vi "Get CFG wrapper.vi"(8 "error in (no error)":errorcluster caption="错误输入（无错误）", 10 "dwCanNodeId":u32, 11 "dwDevIndex":u32) -> (0 "error out":errorcluster caption="错误输出", 1 "UIM_MCFG_INFO_OBJ":T1, 2 "UIM_ICFG_INFO_OBJ":T2, 3 "function return":u32)   [LabVIEW 2016, in "UISimCanFunc_wrapper.lvlib"]
doc: "_declspec (dllexport) DWORD GetCFG_wrapper(DWORD dwDevIndex, DWORD dwCanNodeId,\n P_DUMMY_UIM_ICFG_INFO_OBJ pDummyICFGInfoOut, P_DUMMY_UIM_MCFG_INFO_OBJ pDummyMCFGInfo);"
uses:
  <userlib>/UISimCanFunc_wrapper/UISimCanFunc_wrapper.lvlib
  <userlib>/UISimCanFunc_wrapper/ctl/UIM_ICFG_INFO_OBJ.ctl
  <userlib>/UISimCanFunc_wrapper/ctl/UIM_MCFG_INFO_OBJ.ctl
  <userlib>/UISimCanFunc_wrapper/UISimCanFunc_wrapper.dll
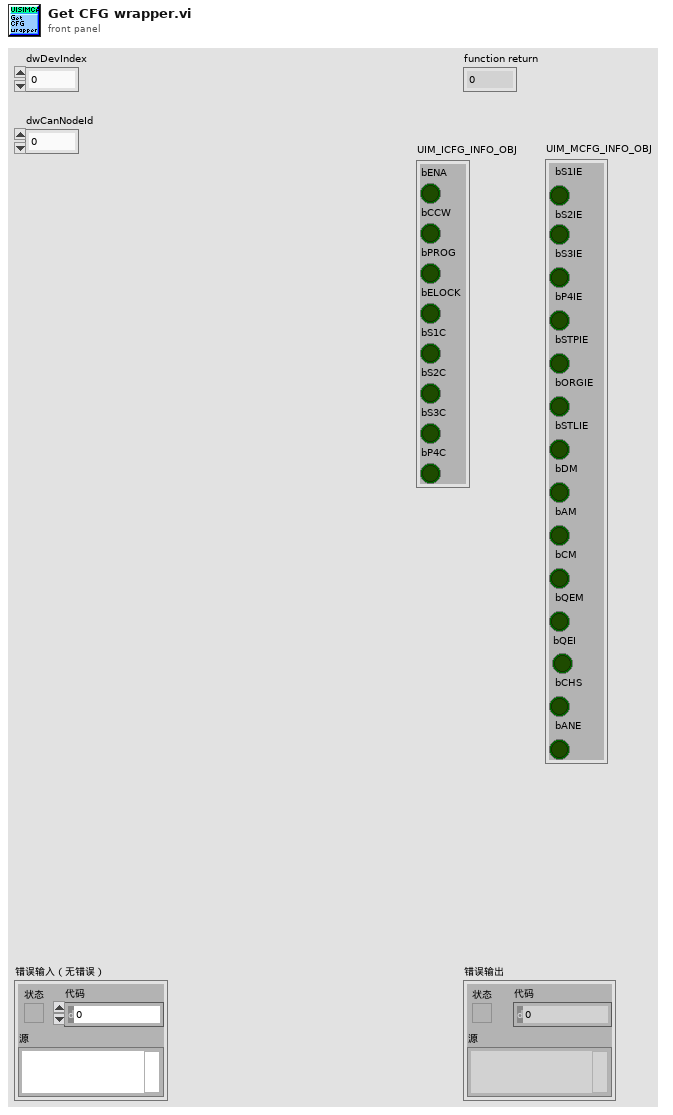
[diagram p1: front panel]
types:
  T1 = typedef "UISimCanFunc_wrapper.lvlib/UIM_MCFG_INFO_OBJ.ctl" = cluster{" bS1IE":bool, " bS2IE":bool, " bS3IE":bool, " bP4IE":bool, " bSTPIE":bool, " bORGIE":bool, " bSTLIE":bool, " bDM":bool, " bAM":bool, " bCM":bool, " bQEM":bool, " bQEI        ":bool, " bCHS":bool, " bANE":bool}
  T2 = typedef "UISimCanFunc_wrapper.lvlib/UIM_ICFG_INFO_OBJ.ctl" = cluster{"bENA":bool, "bCCW":bool, "bPROG":bool, "bELOCK":bool, "bS1C":bool, "bS2C":bool, "bS3C":bool, "bP4C":bool}
  T3 = cluster{"bENA":i32, "bCCW":i32, "bPROG":i32, "bELOCK":i32, "bS1C":i32, "bS2C":i32, "bS3C":i32, "bP4C":i32}
  T4 = cluster{"bS1IE":i32, "bS2IE":i32, "bS3IE":i32, "bP4IE":i32, "bSTPIE":i32, "bORGIE":i32, "bSTLIE":i32, "bDM":i32, "bAM":i32, "bCM":i32, "bQEM":i32, "bQEI":i32, "bCHS":i32, "bANE":i32}
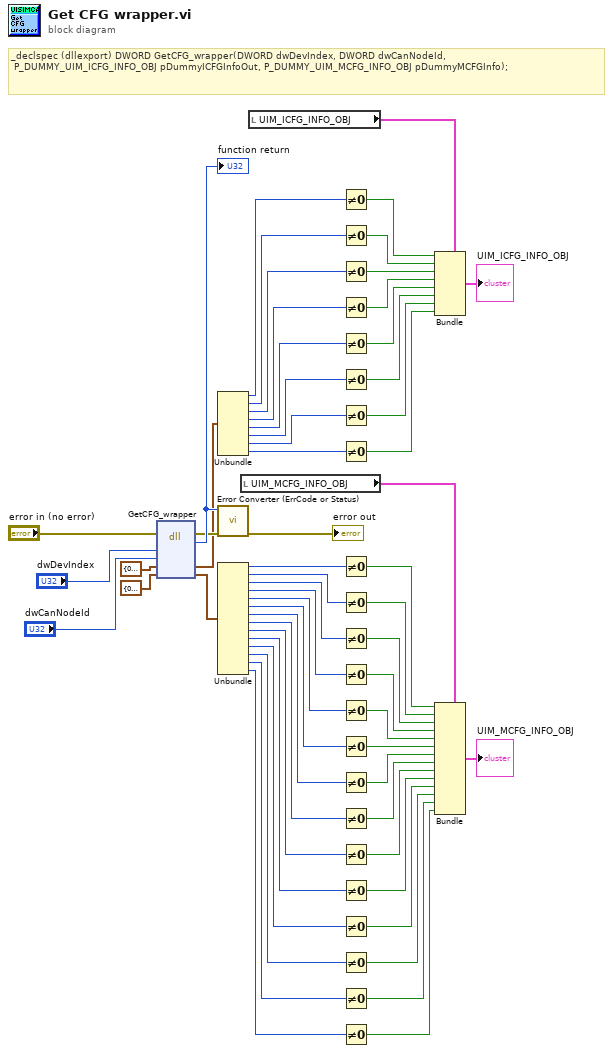
[diagram p0: block diagram]
diagram:
  # "_declspec (dllexport) DWORD GetCFG_wrapper(DWORD dwDevIndex, DWORD dwCanNodeId,\n\tP_DUMMY_UIM_ICFG_INFO_OBJ pDummyICFGInfoOut, P_DUMMY_UIM_MCFG_INFO_OBJ pDummyMCFGInfo);"
  n1 = dll-call lib="C:/Program Files (x86)/National Instruments/LabVIEW 2016/user.lib/UISimCanFunc_wrapper/UISimCanFunc_wrapper.*" fn="GetCFG_wrapper"(error in="error in (no error)", "dwDevIndex"="dwDevIndex", "dwCanNodeId"="dwCanNodeId", "pDummyICFGInfoOut"=T3 {"bENA"=0, "bCCW"=0, "bPROG"=0, "bELOCK"=0, "bS1C"=0, "bS2C"=0, "bS3C"=0, "bP4C"=0}, "pDummyMCFGInfo"=T4 {"bS1IE"=0, "bS2IE"=0, "bS3IE"=0, "bP4IE"=0, "bSTPIE"=0, "bORGIE"=0, "bSTLIE"=0, "bDM"=0, "bAM"=0, "bCM"=0, "bQEM"=0, "bQEI"=0, "bCHS"=0, "bANE"=0}) -> (error out=w54:errorcluster, w58:u32, "pDummyICFGInfoOut"=w1:T3, "pDummyMCFGInfo"=w20:T4)  [unwired: 4 in, 1 out]
  "function return" <- w58
  n2 = Unbundle(w1) -> ("bENA"=w19:i32, "bCCW"=w18:i32, "bPROG"=w17:i32, "bELOCK"=w16:i32, "bS1C"=w11:i32, "bS2C"=w10:i32, "bS3C"=w9:i32, "bP4C"=w8:i32)
  n3 = call <userlib>:"Error Converter (ErrCode or Status).vi"("error in (no error)"=w54, "error code"=w58) -> ("error out"=→"error out":errorcluster)  [unwired: 9 in]
  n4 = Unbundle(w20) -> ("bS1IE"=w50:i32, "bS2IE"=w49:i32, "bS3IE"=w48:i32, "bP4IE"=w47:i32, "bSTPIE"=w46:i32, "bORGIE"=w45:i32, "bSTLIE"=w44:i32, "bDM"=w43:i32, "bAM"=w42:i32, "bCM"=w41:i32, "bQEM"=w40:i32, "bQEI"=w39:i32, "bCHS"=w38:i32, "bANE"=w37:i32)
  n5 = local read "UIM_MCFG_INFO_OBJ"() -> (w21:T1)
  n6 = local read "UIM_ICFG_INFO_OBJ"() -> (w2:T2)
  n7 = Not Equal To 0?(x=w19) -> (x != 0?=w15:bool)
  n8 = Not Equal To 0?(x=w18) -> (x != 0?=w14:bool)
  n9 = Not Equal To 0?(x=w17) -> (x != 0?=w13:bool)
  n10 = Not Equal To 0?(x=w16) -> (x != 0?=w12:bool)
  n11 = Not Equal To 0?(x=w11) -> (x != 0?=w7:bool)
  n12 = Not Equal To 0?(x=w10) -> (x != 0?=w6:bool)
  n13 = Not Equal To 0?(x=w9) -> (x != 0?=w5:bool)
  n14 = Not Equal To 0?(x=w8) -> (x != 0?=w4:bool)
  n15 = Not Equal To 0?(x=w50) -> (x != 0?=w36:bool)
  n16 = Not Equal To 0?(x=w49) -> (x != 0?=w35:bool)
  n17 = Not Equal To 0?(x=w48) -> (x != 0?=w34:bool)
  n18 = Not Equal To 0?(x=w47) -> (x != 0?=w33:bool)
  n19 = Not Equal To 0?(x=w46) -> (x != 0?=w32:bool)
  n20 = Not Equal To 0?(x=w45) -> (x != 0?=w31:bool)
  n21 = Not Equal To 0?(x=w44) -> (x != 0?=w30:bool)
  n22 = Not Equal To 0?(x=w43) -> (x != 0?=w29:bool)
  n23 = Not Equal To 0?(x=w42) -> (x != 0?=w28:bool)
  n24 = Not Equal To 0?(x=w41) -> (x != 0?=w27:bool)
  n25 = Not Equal To 0?(x=w40) -> (x != 0?=w26:bool)
  n26 = Not Equal To 0?(x=w39) -> (x != 0?=w25:bool)
  n27 = Not Equal To 0?(x=w38) -> (x != 0?=w24:bool)
  n28 = Not Equal To 0?(x=w37) -> (x != 0?=w23:bool)
  n29 = Bundle(cluster=w2, "bENA"=w15, "bCCW"=w14, "bPROG"=w13, "bELOCK"=w12, "bS1C"=w7, "bS2C"=w6, "bS3C"=w5, "bP4C"=w4) -> (→"UIM_ICFG_INFO_OBJ":T2)
  n30 = Bundle(cluster=w21, "bS1IE"=w36, "bS2IE"=w35, "bS3IE"=w34, "bP4IE"=w33, "bSTPIE"=w32, "bORGIE"=w31, "bSTLIE"=w30, "bDM"=w29, "bAM"=w28, "bCM"=w27, "bQEM"=w26, "bQEI"=w25, "bCHS"=w24, "bANE"=w23) -> (→"UIM_MCFG_INFO_OBJ":T1)
